vi "Parse Numeric Triple.vi"(8 "error in":errorcluster, 11 "Input String":string) -> (0 "error out":errorcluster, 1 "Value 3":dbl, 2 "Value 2":dbl, 3 "Value 1":dbl)   [LabVIEW 2011]
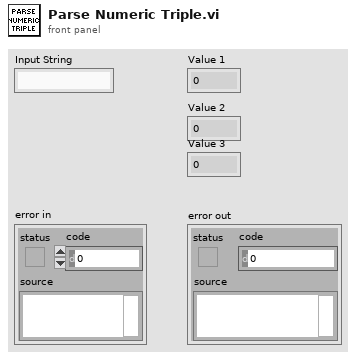
[diagram p1: front panel]
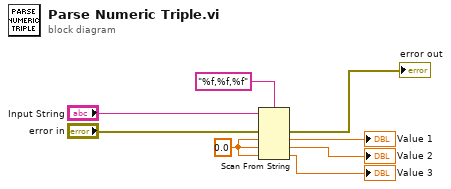
[diagram p0: block diagram]
diagram:
  w7 = 0.0
  n1 = Scan From String(format string="%f,%f,%f", input string="Input String", error in="error in", default 1=w7, default 2=w7, default 3=w7) -> (error out=→"error out":errorcluster, output 1=→"Value 1":dbl, output 2=→"Value 2":dbl, output 3=→"Value 3":dbl)  [unwired: 1 in, 2 out]
